vi "图像填充(子VI).vi"(11 "Image Pixels (U8)":u8[][](array[numeric])) -> (3 "数组":u8[][](array[numeric]))   [LabVIEW 2012]
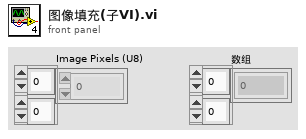
[diagram p1: front panel]
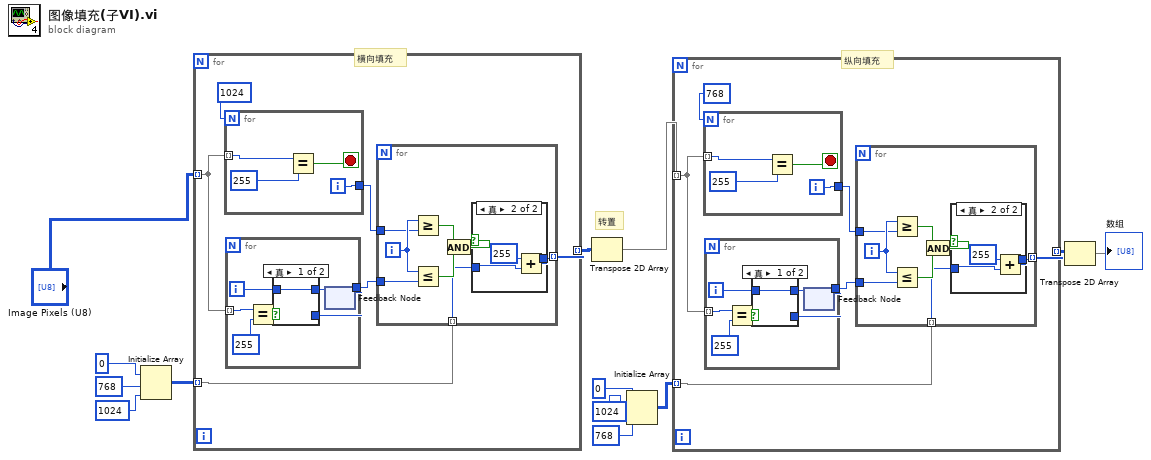
[diagram p0: block diagram]
diagram:
  # "转置"
  # "纵向填充"
  # "横向填充"
  n1 = Initialize Array(u8 0 ("元素"), 768, 1024) -> (w4:u8[][])
  n2 = for {
    tunnel: "Image Pixels (U8)" -> [w18] mode=indexing
    tunnel: w4 -> [w17] mode=indexing
    tunnel: [w16] -> w5 mode=indexing
    n3 = for {
      N: 1024 -> [_]
      tunnel: w18 -> [w40] mode=indexing
      tunnel: [w43] -> w14
      i -> [w43]
      stop <- w41 stop-if-true
      n4 = Equal?(x=w40, y=u8 255) -> (x = y?=w41:bool)
    }
    n5 = for {
      tunnel: w18 -> [w33] mode=indexing
      tunnel: [w35] -> w15
      i -> [w37]
      n6 = Equal?(x=w33, y=u8 255) -> (x = y?=w34:bool)
      n7 = feedback #1() -> (w35:i32)  [unwired: 1 in]
      n8 = case shown="真" w34 {
        tunnel: w37 -> [w38 _]
        tunnel: [w38 w39] -> w36
        tunnel: w35 -> [_ w39]
        frame True {
        }
        frame False {
        }
      }
      n9 = feedback-in #1(w36) -> ()
    }
    n10 = for {
      tunnel: w15 -> [w26]
      tunnel: w17 -> [w21] mode=indexing
      tunnel: [w22] -> w16 mode=indexing
      tunnel: w14 -> [w20]
      i -> [w27]
      n11 = Greater Or Equal?(x=w27, y=w20) -> (x >= y?=w25:bool)
      n12 = Less Or Equal?(x=w27, y=w26) -> (x <= y?=w24:bool)
      n13 = And(x=w25, y=w24) -> (x .and. y?=w23:bool)
      n14 = case shown="真" w23 {
        tunnel: w21 -> [w28 w31]
        tunnel: [w28 w30] -> w22
        frame False {
        }
        frame True {
          n15 = Add(x=u8 255, y=w31) -> (x+y=w30:u8)
        }
      }
    }
  }
  n16 = Transpose 2D Array(2D array=w5) -> (transposed array=w6:u8[][])
  n17 = Initialize Array(u8 0 ("元素"), 1024, 768) -> (w10:u8[][])
  n18 = for {
    tunnel: w6 -> [w48] mode=indexing
    tunnel: w10 -> [w47] mode=indexing
    tunnel: [w46] -> w11 mode=indexing
    n19 = for {
      N: 768 -> [_]
      tunnel: w48 -> [w70] mode=indexing
      tunnel: [w73] -> w44
      i -> [w73]
      stop <- w71 stop-if-true
      n20 = Equal?(x=w70, y=u8 255) -> (x = y?=w71:bool)
    }
    n21 = for {
      tunnel: w48 -> [w63] mode=indexing
      tunnel: [w65] -> w45
      i -> [w67]
      n22 = Equal?(x=w63, y=u8 255) -> (x = y?=w64:bool)
      n23 = feedback #2() -> (w65:i32)  [unwired: 1 in]
      n24 = case shown="真" w64 {
        tunnel: w67 -> [w68 _]
        tunnel: [w68 w69] -> w66
        tunnel: w65 -> [_ w69]
        frame True {
        }
        frame False {
        }
      }
      n25 = feedback-in #2(w66) -> ()
    }
    n26 = for {
      tunnel: w45 -> [w56]
      tunnel: w47 -> [w51] mode=indexing
      tunnel: [w52] -> w46 mode=indexing
      tunnel: w44 -> [w50]
      i -> [w57]
      n27 = Greater Or Equal?(x=w57, y=w50) -> (x >= y?=w55:bool)
      n28 = Less Or Equal?(x=w57, y=w56) -> (x <= y?=w54:bool)
      n29 = And(x=w55, y=w54) -> (x .and. y?=w53:bool)
      n30 = case shown="真" w53 {
        tunnel: w51 -> [w58 w61]
        tunnel: [w58 w60] -> w52
        frame False {
        }
        frame True {
          n31 = Add(x=u8 255, y=w61) -> (x+y=w60:u8)
        }
      }
    }
  }
  n32 = Transpose 2D Array(2D array=w11) -> (transposed array=→"数组":u8[][])
